vi "write_data_to_file.vi"(6 "Titration Points":T4, 7 "Configuration":T1={"Alkalinity Calculation Functions"={"HCl Temp Correction Function"="", "Sample Temp Correction Function"="", "Dosimat Correction Function"="", "Cell Temp Correction Function"="", "HCl Density Function"=""}, "Instrument Settings"={"Relay Port"="COM6", "Agilent Port"="COM5", "Dosimat Port"="COM4", "Thermal Coeffients Path"=path ""}, "Titration Settings"={"Hold Time (sec)"=300, "Initial HCl Increment"=0.0, "Target EMF"=0.0, "Agilent Monitoring Refresh Period"=0.0, "Small HCl Increment"=0.0, "Number of Titration Points"=0}, "Other Settings"={"HCl Concentration"=0.0, "HCl Lot ID"=""}, "Electrode Settings"={"Probe ID - Electrode 1 "=0, "Channel - Electrode 1"=0, "Probe ID - Electrode 2"=0, "Channel - Electrode 2"=0}}, 8 "error in (no error)":errorcluster, 9 "Run Data":T3, 10 "Run Settings":T2, 11 "Path":path) -> (0 "error out":errorcluster)   [LabVIEW 2010]
uses:
  <vilib>/Utility/xml.llb/Read From XML File(string).vi
  <vilib>/Utility/xml.llb/Write to XML File(string).vi
panel:
  # "This control only works when titration is not actively taking place"
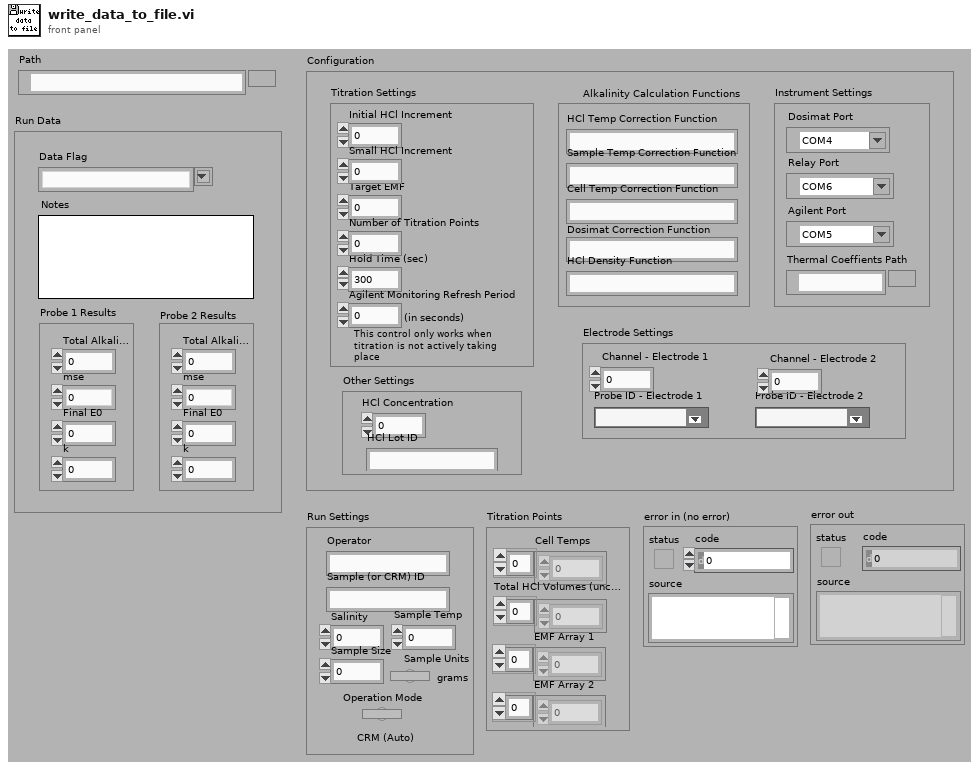
[diagram p1: front panel]
types:
  T1 = cluster{"Alkalinity Calculation Functions":cluster{"HCl Temp Correction Function":string, "Sample Temp Correction Function":string, "Dosimat Correction Function":string, "Cell Temp Correction Function":string, "HCl Density Function":string}, "Instrument Settings":cluster{"Relay Port":refnum<visa-resource-name>, "Agilent Port":refnum<visa-resource-name>, "Dosimat Port":refnum<visa-resource-name>, "Thermal Coeffients Path":path}, "Titration Settings":cluster{"Hold Time (sec)":i16, "Initial HCl Increment":dbl, "Target EMF":dbl, "Agilent Monitoring Refresh Period":dbl, "Small HCl Increment":dbl, "Number of Titration Points":i32}, "Other Settings":cluster{"HCl Concentration":dbl, "HCl Lot ID":string}, "Electrode Settings":cluster{"Probe ID - Electrode 1 ":u16, "Channel - Electrode 1":i32, "Probe ID - Electrode 2":u16, "Channel - Electrode 2":i32}}
  T2 = cluster{"Operator":string, "Sample (or CRM) ID":string, "Sample Temp":dbl, "Salinity":dbl, "Sample Units":bool, "Sample Size":dbl, "Operation Mode":bool}
  T3 = cluster{"Data Flag":string, "Notes":string, "Probe 1 Results":cluster{"Total Alkalinity":dbl, "mse":dbl, "Final E0":dbl, "k":dbl}, "Probe 2 Results":cluster{"Total Alkalinity":dbl, "mse":dbl, "Final E0":dbl, "k":dbl}}
  T4 = cluster{"Cell Temps":dbl[], "Total HCl Volumes (uncorr)":dbl[], "EMF Array 1":dbl[], "EMF Array 2":dbl[]}
  T5 = cluster{"Total Alkalinity":dbl, "mse":dbl, "Final E0":dbl, "k":dbl}
  T6 = enum16{"read", "write crm data", "add electrode"}
  T7 = cluster{"Sample (or CRM) ID":string, "Run Type (Sample or DRM)":string, "Opertator":string, "Data Flag":string, "Salinity":dbl, "Sample Temp":dbl, "Sample Size":dbl, "Sample Units":bool, "Time Completed":timestamp, "Notes":string, "Probe 1 Results":cluster{"Total Alkalinity":dbl, "mse":dbl, "Final E0":dbl, "k":dbl}, "Probe 2 Results":cluster{"Total Alkalinity":dbl, "mse":dbl, "Final E0":dbl, "k":dbl}}
  T8 = cluster{"Time Stamp":timestamp, "Titration Stage":string, "Average Voltage":dbl, "Burette Temp Average":dbl, "Voltage 1":dbl, "Voltage 2":dbl, "Voltage 1 StandDev":dbl, "Voltage 2 StandDev":dbl, "Burette Temp 1":dbl, "Burette Temp 2":dbl, "Cell Temp":dbl, "Acid Temp":dbl, "Room Temp":dbl}[]
  T9 = cluster{"Relay Port":refnum<visa-resource-name>, "Agilent Port":refnum<visa-resource-name>, "Dosimat Port":refnum<visa-resource-name>, "Thermal Coeffients Path":path}
  T10 = cluster{"HCl Concentration":dbl, "HCl Lot ID":string}
  T11 = cluster{"Probe ID - Electrode 1 ":u16, "Channel - Electrode 1":i32, "Probe ID - Electrode 2":u16, "Channel - Electrode 2":i32}
  T12 = cluster{"seconds since 1Jan1904":timestamp, "Operator":string, string, "Sample (or CRM) ID":string, "HCl Lot ID":string, "CRM Alkalinity":dbl, "Salinity":dbl, dbl, dbl, "Probe 1 Results":cluster{"Total Alkalinity":dbl, "mse":dbl, "Final E0":dbl, "k":dbl}, "Probe 2 Results":cluster{"Total Alkalinity":dbl, "mse":dbl, "Final E0":dbl, "k":dbl}}
  T13 = cluster{"Run Data":cluster{"Sample (or CRM) ID":string, "Run Type (Sample or DRM)":string, "Opertator":string, "Data Flag":string, "Salinity":dbl, "Sample Temp":dbl, "Sample Size":dbl, "Sample Units":bool, "Time Completed":timestamp, "Notes":string, "Probe 1 Results":cluster{"Total Alkalinity":dbl, "mse":dbl, "Final E0":dbl, "k":dbl}, "Probe 2 Results":cluster{"Total Alkalinity":dbl, "mse":dbl, "Final E0":dbl, "k":dbl}}, "Configuration":cluster{"Alkalinity Calculation Functions":cluster{"HCl Temp Correction Function":string, "Sample Temp Correction Function":string, "Dosimat Correction Function":string, "Cell Temp Correction Function":string, "HCl Density Function":string}, "Instrument Settings":cluster{"Relay Port":refnum<visa-resource-name>, "Agilent Port":refnum<visa-resource-name>, "Dosimat Port":refnum<visa-resource-name>, "Thermal Coeffients Path":path}, "Titration Settings":cluster{"Hold Time (sec)":i16, "Initial HCl Increment":dbl, "Target EMF":dbl, "Agilent Monitoring Refresh Period":dbl, "Small HCl Increment":dbl, "Number of Titration Points":i32}, "Other Settings":cluster{"HCl Concentration":dbl, "HCl Lot ID":string}, "Electrode Settings":cluster{"Probe ID - Electrode 1 ":u16, "Channel - Electrode 1":i32, "Probe ID - Electrode 2":u16, "Channel - Electrode 2":i32}}, "Agilent Monitoring Record":cluster{"Time Stamp":timestamp, "Titration Stage":string, "Average Voltage":dbl, "Burette Temp Average":dbl, "Voltage 1":dbl, "Voltage 2":dbl, "Voltage 1 StandDev":dbl, "Voltage 2 StandDev":dbl, "Burette Temp 1":dbl, "Burette Temp 2":dbl, "Cell Temp":dbl, "Acid Temp":dbl, "Room Temp":dbl}[], "Titration Points":cluster{"Cell Temps":dbl[], "Total HCl Volumes (uncorr)":dbl[], "EMF Array 1":dbl[], "EMF Array 2":dbl[]}, string}
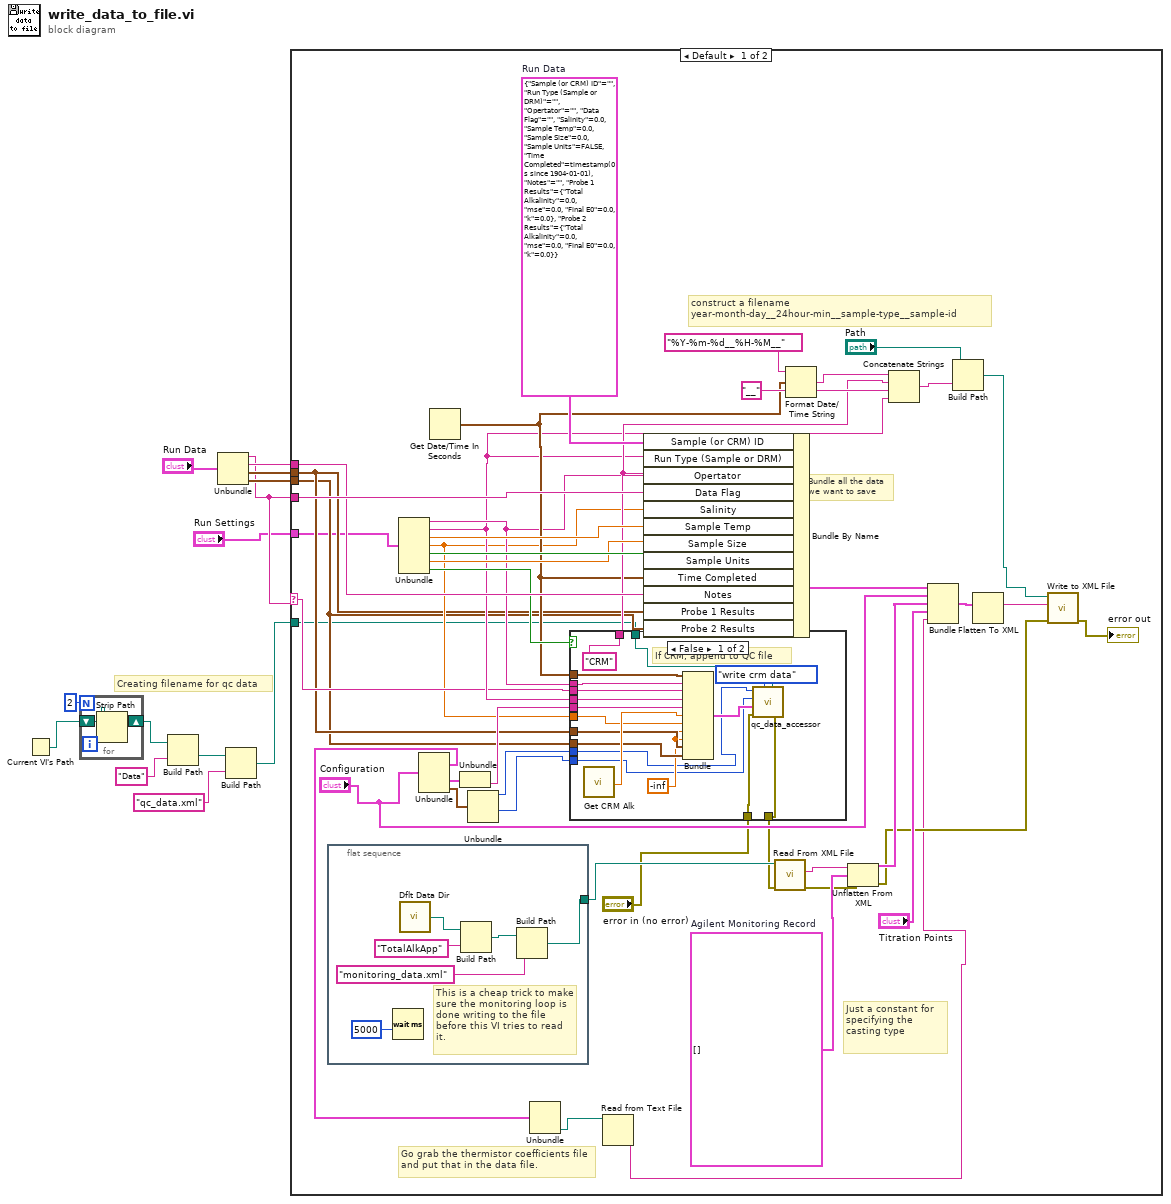
[diagram p0: block diagram]
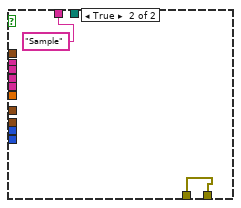
[diagram p2: hidden frame]
diagram:
  # "Creating filename for qc data"
  n1 = Current VI's Path() -> (path=w3:path)
  n2 = for {
    N: 2 -> [_]
    shift-right: [w14] -> w2
    shift-left: w3 -> [w15]
    n3 = Strip Path(path=w15) -> (stripped path=w14:path)  [unwired: 1 out]
  }
  n4 = Build Path(base path=w2, name or relative path="Data") -> (appended path=w5:path)
  n5 = Unbundle("Run Data") -> ("Data Flag"=w9:string, "Notes"=w12:string, "Probe 1 Results"=w11:T5, "Probe 2 Results"=w10:T5)
  n6 = Build Path(base path=w5, name or relative path="qc_data.xml") -> (appended path=w1:path)
  n7 = case shown="Default" w9 {
    selector: w9 -> [w34 _]
    tunnel: w9 -> [w44 _]
    tunnel: w12 -> [w43 _]
    tunnel: w11 -> [w30 _]
    tunnel: w10 -> [w29 _]
    tunnel: "Run Settings" -> [w28 _]
    tunnel: w1 -> [w16 _]
    frame Default {
      w46 = T7 {"Sample (or CRM) ID"="", "Run Type (Sample or DRM)"="", "Opertator"="", "Data Flag"="", "Salinity"=0.0, "Sample Temp"=0.0, "Sample Size"=0.0, "Sample Units"=FALSE, "Time Completed"=timestamp(0 s since 1904-01-01), "Notes"="", "Probe 1 Results"={"Total Alkalinity"=0.0, "mse"=0.0, "Final E0"=0.0, "k"=0.0}, "Probe 2 Results"={"Total Alkalinity"=0.0, "mse"=0.0, "Final E0"=0.0, "k"=0.0}}  # Run Data
      w60 = T8 []  # Agilent Monitoring Record
      # "Go grab the thermistor coefficients file and put that in the data file."
      # "construct a filename \nyear-month-day__24hour-min__sample-type__sample-id"
      # "Bundle all the data we want to save"
      # "Just a constant for specifying the casting type"
      n8 = flat-sequence {
        tunnel: [w83] -> w56
        frame #0 {
          # "This is a cheap trick to make sure the monitoring loop is done writing to the file before this VI tries to read it."
          n9 = Wait (ms)(milliseconds to wait=5000) -> ()  [unwired: 1 out]
          n10 = call <vilib>:"Dflt Data Dir.vi"() -> ("App:Default Data Directory"=w86:path)
          n11 = Build Path(base path=w86, name or relative path="TotalAlkApp") -> (appended path=w84:path)
          n12 = Build Path(base path=w84, name or relative path="monitoring_data.xml") -> (appended path=w83:path)
        }
      }
      n13 = Unbundle(w28) -> ("Operator"=w36:string, "Sample (or CRM) ID"=w35:string, "Sample Temp"=w42:dbl, "Salinity"=w31:dbl, "Sample Units"=w41:bool, "Sample Size"=w40:dbl, "Operation Mode"=w38:bool)
      n14 = Unbundle("Configuration") -> ("Instrument Settings"=w19:T9, "Other Settings"=w33:T10, "Electrode Settings"=w26:T11)  [unwired: 2 out]
      n15 = Get Date/Time In Seconds() -> (seconds since 1Jan1904=w37:timestamp)
      n16 = Unbundle(w33) -> ("HCl Lot ID"=w32:string)  [unwired: 1 out]
      n17 = Unbundle(w26) -> ("Probe ID - Electrode 1"=w25:u16, "Probe ID - Electrode 2"=w24:u16)  [unwired: 2 out]
      n18 = Unbundle(w19) -> ("Thermal Coeffients Path"=w18:path)  [unwired: 3 out]
      n19 = case shown="False" w38 {
        tunnel: ["CRM" "Sample"] -> w39
        tunnel: w37 -> [w77 _]
        tunnel: w36 -> [w76 _]
        tunnel: w35 -> [w75 _]
        tunnel: w34 -> [w74 _]
        tunnel: w32 -> [w73 _]
        tunnel: w31 -> [w70 _]
        tunnel: w30 -> [w69 _]
        tunnel: w29 -> [w68 _]
        tunnel: w25 -> [w66 _]
        tunnel: w24 -> [w65 _]
        tunnel: "error in (no error)" -> [w64 w79]
        tunnel: [w63 w79] -> w20
        tunnel: w16 -> [w61 _]
        frame False {
          w67 = -inf
          # "If CRM, append to QC file"
          n20 = call "Get CRM Alk"() -> ("CRM Alkalinity"=w71:dbl)  [unwired: 17 in, 2 out]
          n21 = Bundle("seconds since 1Jan1904"=w77, "Operator"=w76, w74, "Sample (or CRM) ID"=w75, "HCl Lot ID"=w73, "CRM Alkalinity"=w71, "Salinity"=w70, w67, w67, "Probe 1 Results"=w69, "Probe 2 Results"=w68) -> (w72:T12)  [unwired: 1 in]
          n22 = call "qc_data_accessor.vi"("Path"=w61, "action (open:0)"=T6."write crm data", "error in (no error)"=w64, "CRM Run"=w72, "Electrode 2 Index"=w65, "Electrode 1 Index"=w66) -> ("error out"=w63:errorcluster)  [unwired: 2 in, 3 out]
        }
        frame True {
        }
      }
      n23 = Read from Text File(file (use dialog)=w18) -> (text=w17:string)  [unwired: 3 in, 3 out]
      n24 = Bundle By Name(cluster=w46, "Sample (or CRM) ID"=w35, "Run Type (Sample or DRM)"=w39, "Opertator"=w36, "Data Flag"=w44, "Salinity"=w31, "Sample Temp"=w42, "Sample Size"=w40, "Sample Units"=w41, "Time Completed"=w37, "Notes"=w43, "Probe 1 Results"=w30, "Probe 2 Results"=w29) -> (w45:T7)
      n25 = call-poly <vilib>:"Read From XML File.vi"("error in (no error)"=w20, "XML File Path"=w56) -> ("error out"=w58:errorcluster, "XML Elements"=w59:string)  [unwired: 7 in, 1 out]
      n26 = Format Date/Time String(time format string (%c)="%Y-%m-%d__%H-%M__", seconds (now)=w37) -> (date/time string=w52:string)  [unwired: 1 in]
      n27 = Unflatten From XML(xml string=w59, type=w60, error in (no error)=w58) -> (value=w57:T8, error out=w23:errorcluster)
      n28 = Concatenate Strings(w52, w39, "__", w35) -> (w49:string)
      n29 = Bundle("Run Data"=w45, "Configuration"="Configuration", "Agilent Monitoring Record"=w57, "Titration Points"="Titration Points", w17) -> (w55:T13)  [unwired: 1 in]
      n30 = Build Path(base path="Path", name or relative path=w49) -> (appended path=w47:path)
      n31 = Flatten To XML(anything=w55) -> (xml string=w54:string)
      n32 = call-poly <vilib>:"Write to XML File.vi"("error in (no error)"=w23, "XML Input"=w54, "XML File Path"=w47) -> ("error out"=→"error out":errorcluster)  [unwired: 6 in, 2 out]
    }
    frame "Don't Save Data" {
    }
  }
